vi "station2_bit to array .vi"(8 "error in (no error)":errorcluster, 11 "ST1_Controls_from_PLC":i64[](array[numeric])=[0, 0, 0, 0, 0]) -> (0 "error out":errorcluster, 2 "1 on state":i32[](array[numeric]), 3 "1 result array":bool[](array[boolean]))   [LabVIEW 2017]
panel:
  out "fpl st2":bool
  out "LB st2":bool
  out "cycle rslt stn 2":bool
  out "HB st2":bool
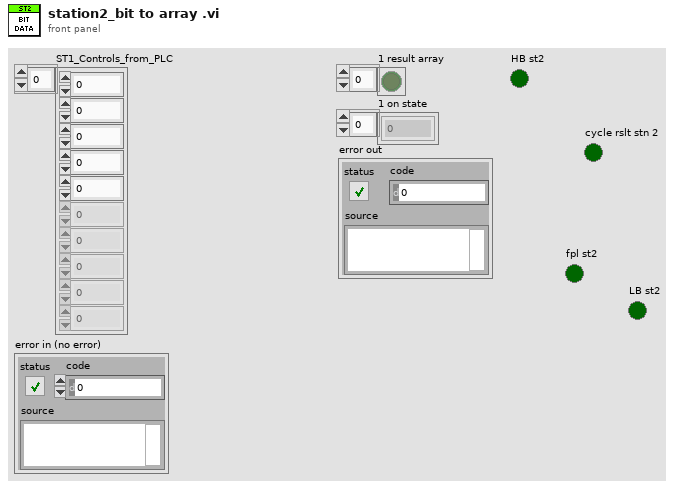
[diagram p1: front panel]
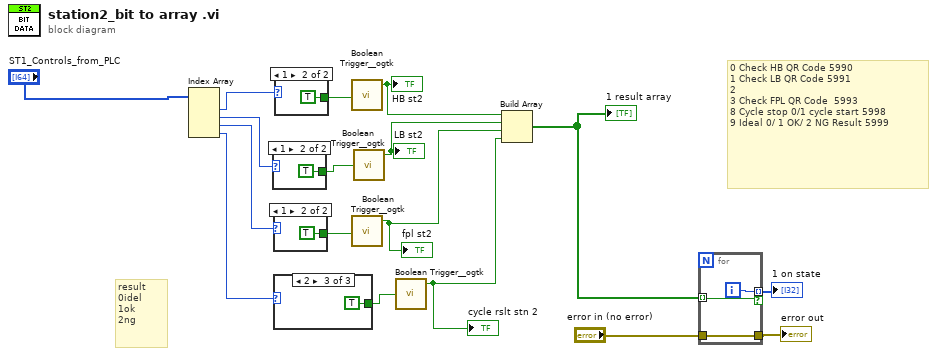
[diagram p0: block diagram]
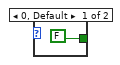
[diagram p2: hidden frame]
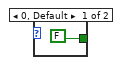
[diagram p3: hidden frame]
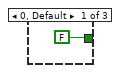
[diagram p4: hidden frame]
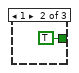
[diagram p5: hidden frame]
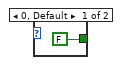
[diagram p6: hidden frame]
diagram:
  # "0 Check HB QR Code 5990\n1 Check LB QR Code 5991\n2 \n3 Check FPL QR Code  5993 \n8 Cycle stop 0/1 cycle start 5998 \n9 Ideal 0/ 1 OK/ 2 NG Result 5999"
  # "result\n0idel\n1ok\n2ng"
  n1 = Index Array(array="ST1_Controls_from_PLC") -> (element #1=w17:i64, element #2=w5:i64, element #3=w6:i64, element #4=w4:i64)  [unwired: 4 in]
  n2 = case shown="1" w5 {
    tunnel: [FALSE TRUE] -> w8
    frame 0, Default {
    }
    frame 1 {
    }
  }
  n3 = case shown="1" w6 {
    tunnel: [FALSE TRUE] -> w7
    frame 0, Default {
    }
    frame 1 {
    }
  }
  n4 = case shown="2" w4 {
    tunnel: [FALSE TRUE TRUE] -> w16
    frame 0, Default {
    }
    frame 1 {
    }
    frame 2 {
    }
  }
  n5 = case shown="1" w17 {
    tunnel: [FALSE TRUE] -> w15
    frame 0, Default {
    }
    frame 1 {
    }
  }
  n6 = call <userlib>:"Boolean Trigger__ogtk.vi"("Boolean Input"=w15) -> ("Rising Edge"=w13:bool)  [unwired: 1 in, 1 out]
  "HB st2" <- w13
  n7 = call <userlib>:"Boolean Trigger__ogtk.vi"("Boolean Input"=w7) -> ("Rising Edge"=w2:bool)  [unwired: 1 in, 1 out]
  "fpl st2" <- w2
  n8 = call <userlib>:"Boolean Trigger__ogtk.vi"("Boolean Input"=w8) -> ("Rising Edge"=w3:bool)  [unwired: 1 in, 1 out]
  "LB st2" <- w3
  n9 = call <userlib>:"Boolean Trigger__ogtk.vi"("Boolean Input"=w16) -> ("Rising Edge"=w1:bool)  [unwired: 1 in, 1 out]
  "cycle rslt stn 2" <- w1
  n10 = Build Array(w13, w3, w2, w1) -> (w12:bool[])
  "1 result array" <- w12
  n11 = for {
    tunnel: [w29] -> w11 mode=indexing if=w27
    tunnel: "error in (no error)" -> [w28]
    tunnel: [w28] -> w10
    tunnel: w12 -> [w27] mode=indexing
    i -> [w29]
  }
  "1 on state" <- w11
  "error out" <- w10
